vi "Autonomous Independent.vi"() -> ()   [LabVIEW 2011]
doc: "This VI is called when autonomous begins, and will automatically be terminated when autonomous ends. You can carry out timed or sensor driven robot movement independently without needing to return to the caller."
uses:
  Robot Global Data.vi
panel:
  in  "Record Auton":bool
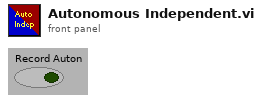
[diagram p1: front panel]
types:
  T1 = typedef "WPI_MotorControlDeviceRef.ctl" = cluster{"DeviceStatus":errorcluster, "Type":enum16{"PWM", "CAN"}, "PWM":cluster{"Digital Module":T2, "PWM Channel":T3, "DeadBand":T4}, "CAN":cluster{"Device Number":u8, "Control Mode":T5, "Semaphore":T6, "Max Vout":dbl}, "Invert":bool, "TransformRef":T7, "InvTransformRef":T7}
  T2 = typedef "FPGA_TypedefDigitalModule.ctl" = enum16{"Digital Module 1", "Digital Module 2"}
  T3 = typedef "FPGA_DIOPWMChannel.ctl" = enum8{"PWM 1", "PWM 2", "PWM 3", "PWM 4", "PWM 5", "PWM 6", "PWM 7", "PWM 8", "PWM 9", "PWM 10", "Invalid"}
  T4 = typedef "WPI_PWMDeadband.ctl" = cluster{"Name":string, "maxPositivePwm":i32, "minPositivePwm":i32, "centerPwm":i32, "maxNegativePwm":i32, "minNegativePwm":i32, "angularRange":u16}
  T5 = typedef "WPI_CANJaguar_ControlMode.ctl" = enum8{"Percent VBus", "Current", "Speed", "Position", "Voltage"}
  T6 = typedef "Semaphore RefNum" = refnum<k1>
  T7 = typedef "WPI_PWMTransform_ConPane.ctl" = refnum<vi>
  T8 = typedef "WPI_ServoDeviceRef.ctl" = cluster{"DeviceStatus":errorcluster, "Digital Module":T2, "PWM Channel":T3, "DeadBand":T4}
  T9 = typedef "WPI_EncoderDevRef.ctl" = cluster{"DevStatus":errorcluster, "EncoderIndex":T10, "CounterIndex":T11, "DistancePerCount":dbl, "Decoding Type":T12}
  T10 = typedef "FPGA_EncoderIdx.ctl" = enum8{"Enc 0", "Enc 1", "Enc 2", "Enc 3", "Invalid"}
  T11 = typedef "FPGA_CounterCtrSystemIndex.ctl" = enum8{"Ctr 0", "Ctr 1", "Ctr 2", "Ctr 3", "Ctr 4", "Ctr 5", "Ctr 6", "Ctr 7", "Invalid"}
  T12 = typedef "WPI_EncoderType.ctl" = enum16{"1x", "2x", "4x"}
  T13 = typedef "WPI_GyroDevRef.ctl" = cluster{"DevStatus":errorcluster, "Analog Module":T14, "Analog Channel":T15, "Offset":dbl, "Gain (VoltsPerDegree/Second)":dbl}
  T14 = typedef "FPGA_TypedefAnalogModule.ctl" = enum16{"Analog Module 1", "Analog Module 2"}
  T15 = typedef "FPGA_AIChannel.ctl" = enum8{"AI 1", "AI 2", "AI 3", "AI 4", "AI 5", "AI 6", "AI 7", "AI 8", "Invalid"}
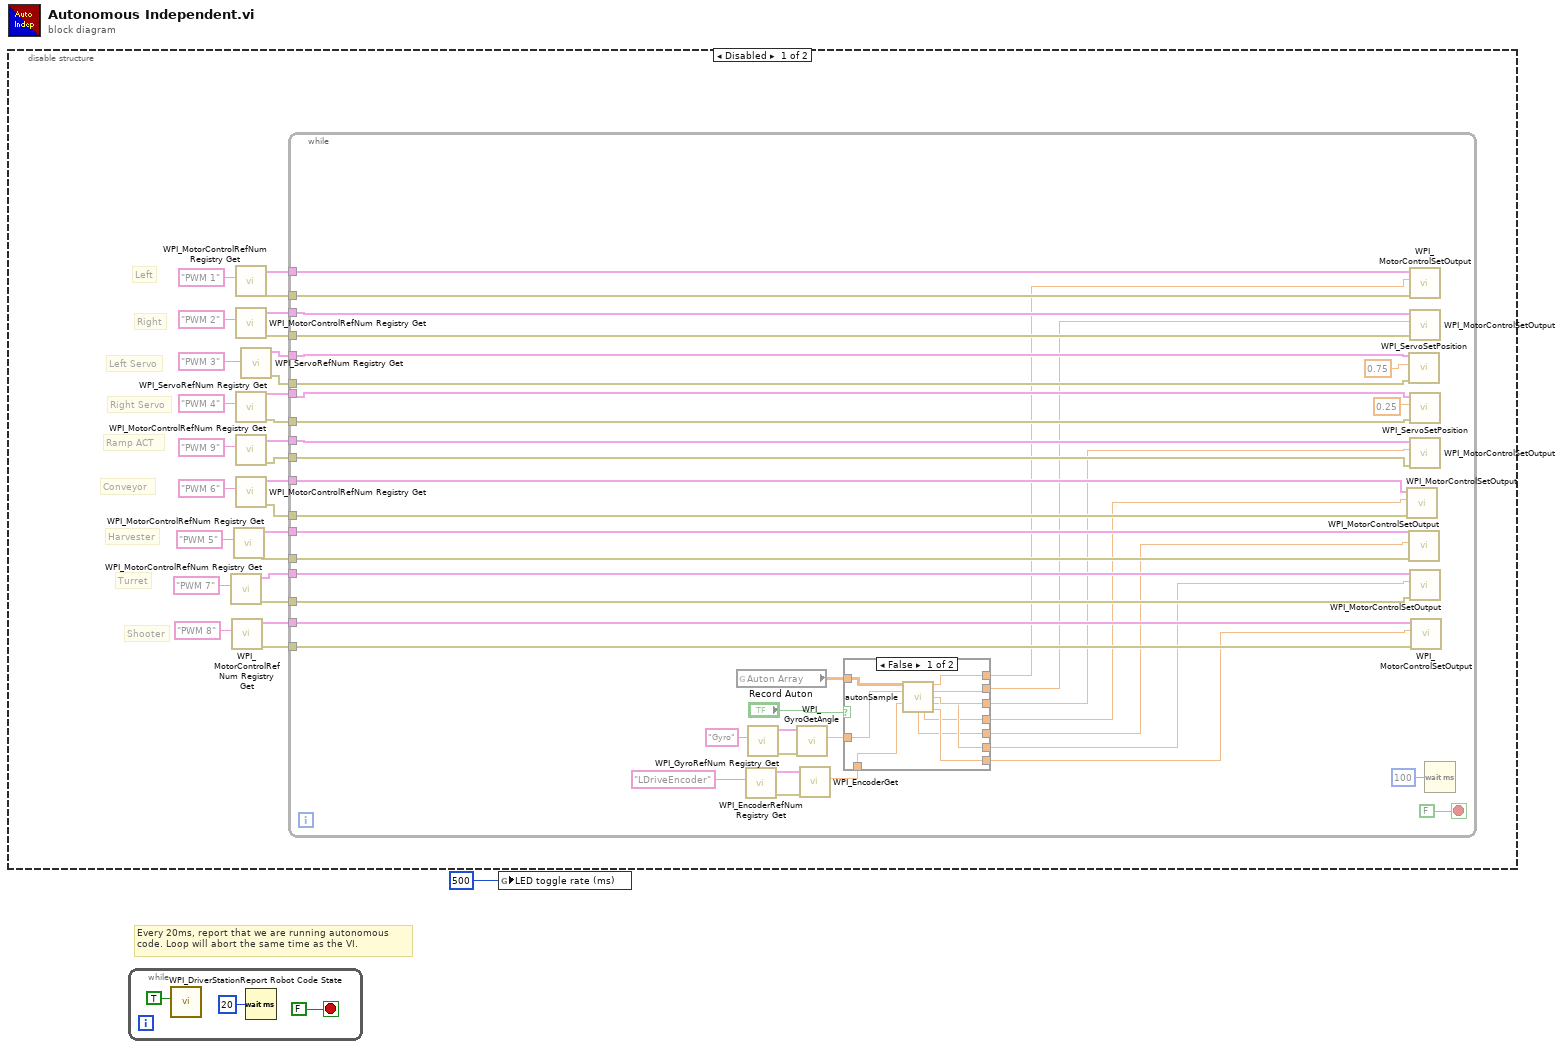
[diagram p0: block diagram]
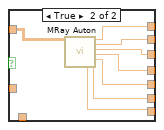
[diagram p2: hidden frame]
diagram:
  # "Every 20ms, report that we are running autonomous\ncode. Loop will abort the same time as the VI."
  n1 = disable-structure shown="Disabled" {
    frame Disabled {
      # "Shooter"
      # "Turret"
      # "Conveyor"
      # "Harvester"
      # "Ramp ACT"
      # "Right Servo"
      # "Left Servo"
      # "Right"
      # "Left"
      n2 = call <vilib>:"WPI_MotorControlRefNum Registry Get.vi"("refnum name"="PWM 7") -> ("error out"=w9:errorcluster, "MotorControlDevRef"=w10:T1)  [unwired: 9 in]
      n3 = call <vilib>:"WPI_MotorControlRefNum Registry Get.vi"("refnum name"="PWM 8") -> ("error out"=w7:errorcluster, "MotorControlDevRef"=w8:T1)  [unwired: 9 in]
      n4 = call <vilib>:"WPI_MotorControlRefNum Registry Get.vi"("refnum name"="PWM 5") -> ("error out"=w11:errorcluster, "MotorControlDevRef"=w12:T1)  [unwired: 9 in]
      n5 = call <vilib>:"WPI_MotorControlRefNum Registry Get.vi"("refnum name"="PWM 1") -> ("error out"=w2:errorcluster, "MotorControlDevRef"=w24:T1)  [unwired: 9 in]
      n6 = call <vilib>:"WPI_MotorControlRefNum Registry Get.vi"("refnum name"="PWM 2") -> ("error out"=w3:errorcluster, "MotorControlDevRef"=w23:T1)  [unwired: 9 in]
      n7 = call <vilib>:"WPI_ServoRefNum Registry Get.vi"("refnum name"="PWM 4") -> ("error out"=w5:errorcluster, "ServoDeviceRef"=w22:T8)  [unwired: 9 in]
      n8 = call <vilib>:"WPI_MotorControlRefNum Registry Get.vi"("refnum name"="PWM 9") -> ("error out"=w6:errorcluster, "MotorControlDevRef"=w21:T1)  [unwired: 9 in]
      n9 = call <vilib>:"WPI_MotorControlRefNum Registry Get.vi"("refnum name"="PWM 6") -> ("error out"=w16:errorcluster, "MotorControlDevRef"=w17:T1)  [unwired: 9 in]
      n10 = call <vilib>:"WPI_ServoRefNum Registry Get.vi"("refnum name"="PWM 3") -> ("error out"=w4:errorcluster, "ServoDeviceRef"=w19:T8)  [unwired: 9 in]
      n11 = while {
        tunnel: w24 -> [w65]
        tunnel: w23 -> [w64]
        tunnel: w19 -> [w59]
        tunnel: w22 -> [w60]
        tunnel: w21 -> [w63]
        tunnel: w17 -> [w58]
        tunnel: w16 -> [w57]
        tunnel: w12 -> [w56]
        tunnel: w11 -> [w55]
        tunnel: w10 -> [w54]
        tunnel: w9 -> [w53]
        tunnel: w8 -> [w52]
        tunnel: w7 -> [w51]
        tunnel: w6 -> [w50]
        tunnel: w5 -> [w49]
        tunnel: w4 -> [w48]
        tunnel: w3 -> [w47]
        tunnel: w2 -> [w46]
        stop <- FALSE stop-if-true
        n12 = global read "Robot Global Data.vi" "Auton Array"() -> (w44:dbl[][])
        n13 = call <vilib>:"WPI_EncoderRefNum Registry Get.vi"("refnum name"="LDriveEncoder") -> ("error out"=w41:errorcluster, "EncoderDevRef"=w42:T9)  [unwired: 9 in]
        n14 = call <vilib>:"WPI_GyroRefNum Registry Get.vi"("refnum name"="Gyro") -> ("error out"=w39:errorcluster, "GyroDevRef"=w40:T13)  [unwired: 9 in]
        n15 = call <vilib>:"WPI_GyroGetAngle.vi"("error in (no error)"=w39, "GyroDevRef"=w40) -> ("Angle"=w37:dbl)  [unwired: 6 in, 3 out]
        n16 = call <vilib>:"WPI_EncoderGet.vi"("error in (no error)"=w41, "EncoderDevRef"=w42) -> ("Distance"=w36:dbl)  [unwired: 4 in, 5 out]
        n17 = case shown="False" "Record Auton" {
          tunnel: w44 -> [w77 w85]
          tunnel: w37 -> [w76 _]
          tunnel: w36 -> [w75 _]
          tunnel: [w74 w84] -> w35
          tunnel: [w73 w83] -> w34
          tunnel: [w72 w82] -> w33
          tunnel: [w69 w81] -> w32
          tunnel: [w68 w80] -> w31
          tunnel: [w71 w79] -> w30
          tunnel: [w70 w78] -> w29
          frame False {
            n18 = call "autonSample.vi"("Auton Array"=w77, "MeasuredHeading"=w76, "EncoderDistance"=w75) -> ("Left Drive"=w74:dbl, "Right Drive"=w73:dbl, "Ramp ACT motor"=w72:dbl, "Turret Rotation"=w71:dbl, "Conveyor"=w68:dbl, "Harvester"=w69:dbl, "Shooter motor output"=w70:dbl)  [unwired: 6 in]
          }
          frame True {
            n19 = call "MRay Auton.vi"("Auton Array"=w85) -> ("Shooter"=w78:dbl, "Left Drive"=w84:dbl, "Right Drive"=w83:dbl, "Ramp ACT motor"=w82:dbl, "Conveyor"=w81:dbl, "Harvester"=w80:dbl, "Turret Rotation"=w79:dbl)  [unwired: 12 in]
          }
        }
        n20 = call <vilib>:"WPI_MotorControlSetOutput.vi"("error in (no error)"=w57, "Output"=w32, "MotorControlDevRef"=w58) -> ()  [unwired: 7 in, 2 out]
        n21 = call <vilib>:"WPI_ServoSetPosition.vi"("error in (no error)"=w48, "Position"=0.75 ("Output"), "ServoDeviceRef"=w59) -> ()  [unwired: 7 in, 2 out]
        n22 = call <vilib>:"WPI_MotorControlSetOutput.vi"("error in (no error)"=w55, "Output"=w31, "MotorControlDevRef"=w56) -> ()  [unwired: 7 in, 2 out]
        n23 = call <vilib>:"WPI_MotorControlSetOutput.vi"("error in (no error)"=w46, "Output"=w35, "MotorControlDevRef"=w65) -> ()  [unwired: 7 in, 2 out]
        n24 = call <vilib>:"WPI_MotorControlSetOutput.vi"("error in (no error)"=w47, "Output"=w34, "MotorControlDevRef"=w64) -> ()  [unwired: 7 in, 2 out]
        n25 = call <vilib>:"WPI_ServoSetPosition.vi"("error in (no error)"=w49, "Position"=0.25 ("Output"), "ServoDeviceRef"=w60) -> ()  [unwired: 7 in, 2 out]
        n26 = call <vilib>:"WPI_MotorControlSetOutput.vi"("error in (no error)"=w50, "Output"=w33, "MotorControlDevRef"=w63) -> ()  [unwired: 7 in, 2 out]
        n27 = call <vilib>:"WPI_MotorControlSetOutput.vi"("error in (no error)"=w53, "Output"=w30, "MotorControlDevRef"=w54) -> ()  [unwired: 7 in, 2 out]
        n28 = call <vilib>:"WPI_MotorControlSetOutput.vi"("error in (no error)"=w51, "Output"=w29, "MotorControlDevRef"=w52) -> ()  [unwired: 7 in, 2 out]
        n29 = Wait (ms)(milliseconds to wait=u32 100) -> ()  [unwired: 1 out]
      }
    }
    frame Enabled {
    }
  }
  n30 = while {
    stop <- FALSE stop-if-true
    n31 = call <vilib>:"WPI_DriverStationReport Robot Code State.vi"("Autonomous"=TRUE) -> ()  [unwired: 10 in, 1 out]
    n32 = Wait (ms)(milliseconds to wait=u32 20) -> ()  [unwired: 1 out]
  }
  n33 = global write "Robot Global Data.vi" "LED toggle rate (ms)"(u32 500 ("LED ms toggle rate")) -> ()
